vi "Get Type Specializations.vi"(8 "error in":errorcluster, 11 "measurement plugin service in":refnum<class "Measurement Plugin Service.lvclass">) -> (0 "error out":errorcluster, 2 "type specializations":T1[](array[typedef]), 3 "measurement plugin service out":refnum<class "Measurement Plugin Service.lvclass">)   [LabVIEW 2020, in "Measurement Plugin Measurement Server.lvlib" / "Measurement Plugin Service.lvclass"]
uses:
  Measurement Plugin Service.lvclass
  Helpers/TypeDefs/Parameter Type Specialization.ctl
  Helpers/TypeDefs/Type Specialization.ctl
  Helpers/TypeDefs/Type Specialization Key.ctl
  Measurement Plugin Measurement Server.lvlib
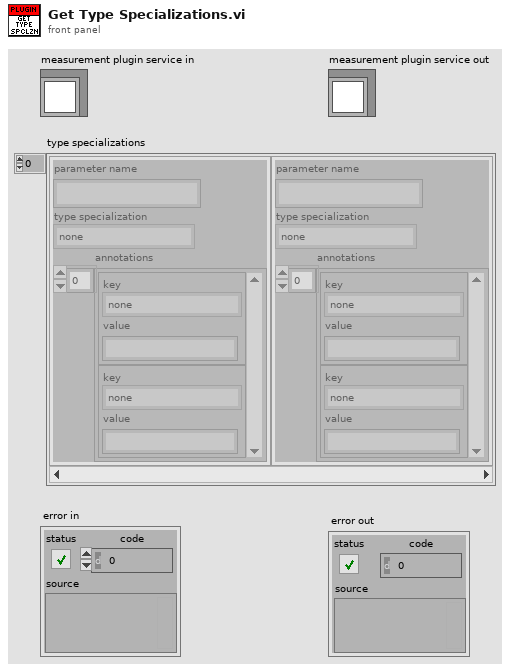
[diagram p1: front panel]
types:
  T1 = typedef "Measurement Plugin Measurement Server.lvlib/Parameter Type Specialization.ctl" = cluster{"parameter name":string, "type specialization":T2, "annotations":cluster{"key":T3, "value":string}[]}
  T2 = typedef "Measurement Plugin Measurement Server.lvlib/Type Specialization.ctl" = enum16{"none", "pin", "path", "enum", "ioresource"}
  T3 = typedef "Measurement Plugin Measurement Server.lvlib/Type Specialization Key.ctl" = enum16{"none", "pin.instrument_type", "enum.values", "ioresource.instrument_type"}
  T4 = typedef "Measurement Plugin Measurement Server.lvlib/Measurement Plugin Service.lvclass/Plugin Paths.ctl" = cluster{"get measurement details VI path":path, "get type specializations VI path":path, "get UI details VI path":path, "measurement logic VI path":path, "measurement configuration ctl path":path, "measurement results ctl path":path}
  T5 = typedef "MeasurementLink Measurement Server.lvlib/Parameter Type Specialization.ctl" = cluster{"parameter name":string, "type specialization":T6, "annotations":cluster{"key":T7, "value":string}[]}
  T6 = typedef "MeasurementLink Measurement Server.lvlib/Type Specialization.ctl" = enum16{"none", "pin", "path", "enum", "ioresource"}
  T7 = typedef "MeasurementLink Measurement Server.lvlib/Type Specialization Key.ctl" = enum16{"none", "pin.instrument_type", "enum.values", "ioresource.instrument_type"}
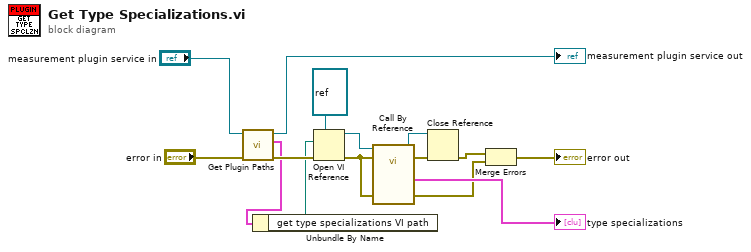
[diagram p0: block diagram]
diagram:
  n1 = call-dynamic "Get Plugin Paths.vi"("error in"="error in", "measurement plugin service in"="measurement plugin service in") -> ("error out"=w9:errorcluster, "plugin paths"=w1:T4, "measurement plugin service out"=→"measurement plugin service out":refnum<class "Measurement Plugin Service.lvclass">)  [unwired: 7 in]
  n2 = Unbundle By Name(w1) -> ("get type specializations VI path"=w8:path)
  n3 = Open VI Reference(type specifier VI Refnum (for type only)=refnum<vi> refnum, vi path=w8, error in (no error)=w9) -> (vi reference=w12:refnum<vi>, error out=w6:errorcluster)  [unwired: 3 in]
  n4 = call-by-ref "?"(reference=w12, error in=w6, "error in"=w6) -> (reference out=w11:refnum<vi>, error out=w10:errorcluster, 0:"error out"=w2:errorcluster, "type specializations"=→"type specializations":T5[])  [unwired: 9 in]
  n5 = Close Reference(reference=w11, error in (no error)=w10) -> (error out=w4:errorcluster)
  n6 = Merge Errors(w4, w2) -> (→"error out":errorcluster)
